vi "BuildFileText.vi"(11 "Code":string) -> (2 "to send":string, 3 "commands":string[](array[string]))   [LabVIEW 2022 SP3]
uses:
  <vilib>/Utility/error.llb/Trim Whitespace One-Sided.vi
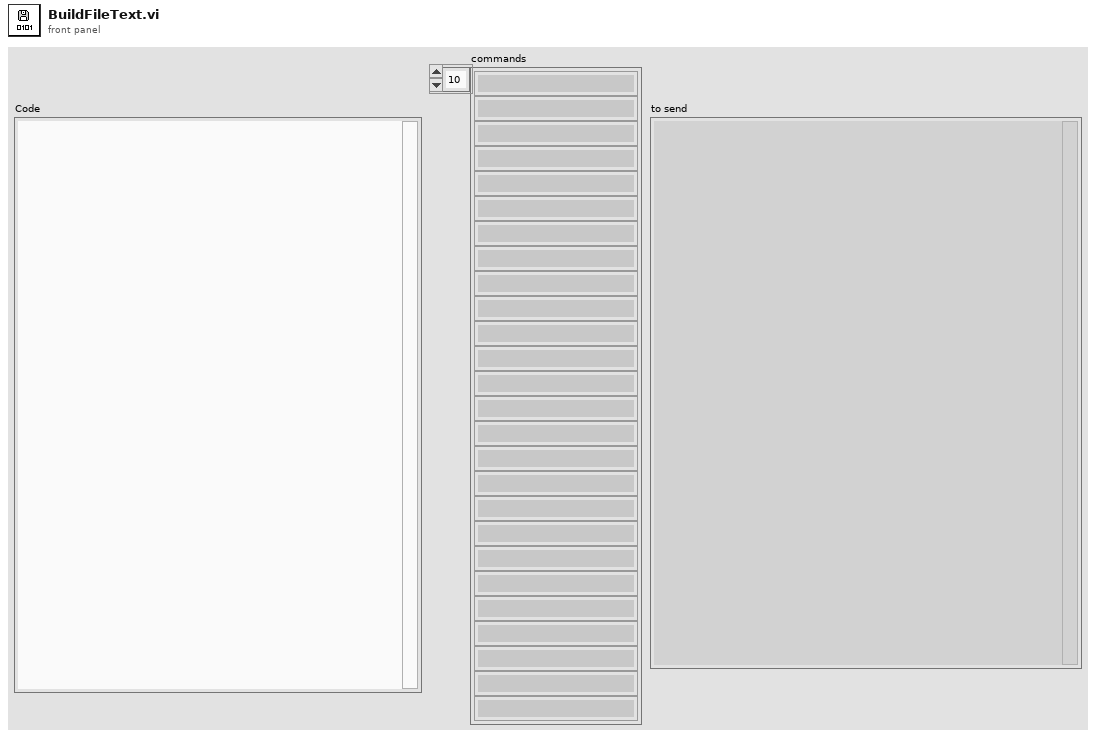
[diagram p1: front panel]
types:
  T1 = typedef "Preferences.ctl" = cluster{"python":string, "arduino CLI":path, "pythonCodes":cluster{"pythonCode":path, "Color":u32}[], "FontSize":u8, "Text Colors":cluster{"Quote":u32, "function":u32, "Python":u32, "Comment":u32, "Triple Quote":u32, "Text":u32}, "SSH Logins":cluster{"IP Address":string, "Username":string, "password":string}[], "packet size":u8}
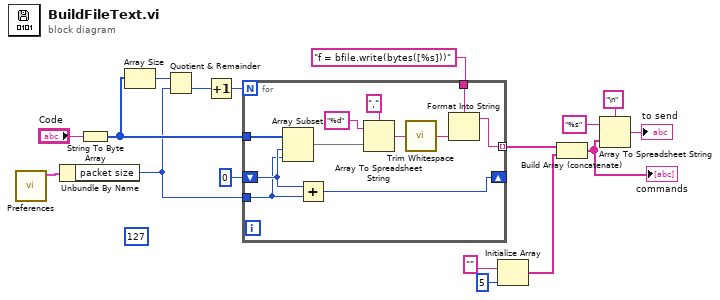
[diagram p0: block diagram]
diagram:
  (unwired) 127 ("length (rest)")
  n1 = call "Preferences.vi"() -> ("Preferences out"=w2:T1)  [unwired: 10 in, 1 out]
  n2 = Unbundle By Name(w2) -> ("packet size"=w1:u8)
  n3 = String To Byte Array(string="Code") -> (unsigned byte array=w15:u8[])
  n4 = Array Size(array=w15) -> (size(s)=w8:i32)
  n5 = Quotient & Remainder(x=w8, y=w1) -> (floor(x/y)=w9:i32)  [unwired: 1 out]
  n6 = Increment(x=w9) -> (x+1=w16:i32)
  n7 = for {
    N: w16 -> [_]
    shift-right: [w27] -> _
    shift-left: 0 -> [w28]
    tunnel: w1 -> [w26]
    tunnel: w15 -> [w25]
    tunnel: [w20] -> w14 mode=indexing
    tunnel: "f = bfile.write(bytes([%s]))" -> [w18]
    n8 = Array Subset(array=w25, index=w28, length=w26) -> (w21:u8[])
    n9 = Add(x=w28, y=w26) -> (x+y=w27:i32)
    n10 = Array To Spreadsheet String(delimiter (Tab)=",", array=w21, 3:"%d" ("format string")) -> (spreadsheet string=w22:string)
    n11 = call <vilib>:"Trim Whitespace.vi"("string"=w22) -> ("trimmed string"=w19:string)  [unwired: 1 in]
    n12 = Format Into String(format string=w18, w19) -> (resulting string=w20:string)  [unwired: 2 in, 1 out]
  }
  n13 = Initialize Array("" ("delimiter (Tab)"), 5 ("dimension size")) -> (w4:string[])
  n14 = Build Array (concatenate)(w14, w4) -> (w10:string[])
  "commands" <- w10
  n15 = Array To Spreadsheet String(delimiter (Tab)="\n", array=w10, 3:"%s" ("format string")) -> (spreadsheet string=→"to send":string)
